vi "filter8.vi"(6 "initialize":bool, 8 "sampling freq: fs":dbl=1000.0 format="%#_13g", 9 "low cutoff freq: fl":dbl=30.0 format="%0.3f", 11 "X":dbl[](array[numeric])) -> (3 "Filtered X":dbl[](array[numeric]))   [LabVIEW 2016]
uses:
  <vilib>/imath/engines/lvmath2/RunTimeEngine/ErrorHandling/NIMS_Finalize Error.vi
  <vilib>/imath/engines/lvmath2/RunTimeEngine/NodeEndStatement/NIMS_NodeEndStatement_Output.vi
  <instcachedir>/0/NIMS_NodeEndStatement_Output_53EC0D466D134D7ABD903AC30B43404B.lvgen/NIMS_NodeEndStatement_Output_53EC0D466D134D7ABD903AC30B43404B_005.vi
  <vilib>/imath/engines/lvmath2/RunTimeEngine/BuiltInFunctions/double/NIMS_double.vi
  <instcachedir>/0/NIMS_double_34E32F64C2B04A25A042F4CA881A0A41.lvgen/NIMS_double_34E32F64C2B04A25A042F4CA881A0A41_002.vi
  <vilib>/ptbypt/NI_PtbyPt.lvlib
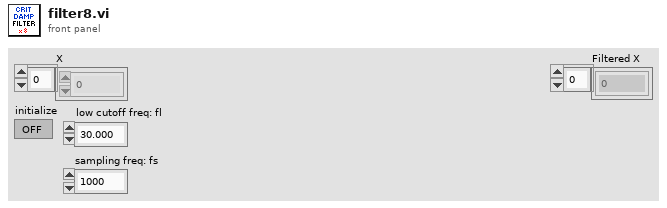
[diagram p1: front panel]
types:
  T1 = cluster{"filter structure":enum32{"IIR 2nd Order", "IIR 4th Order"}, "Reverse Coefficients":dbl[], "Forward Coefficients":dbl[]}
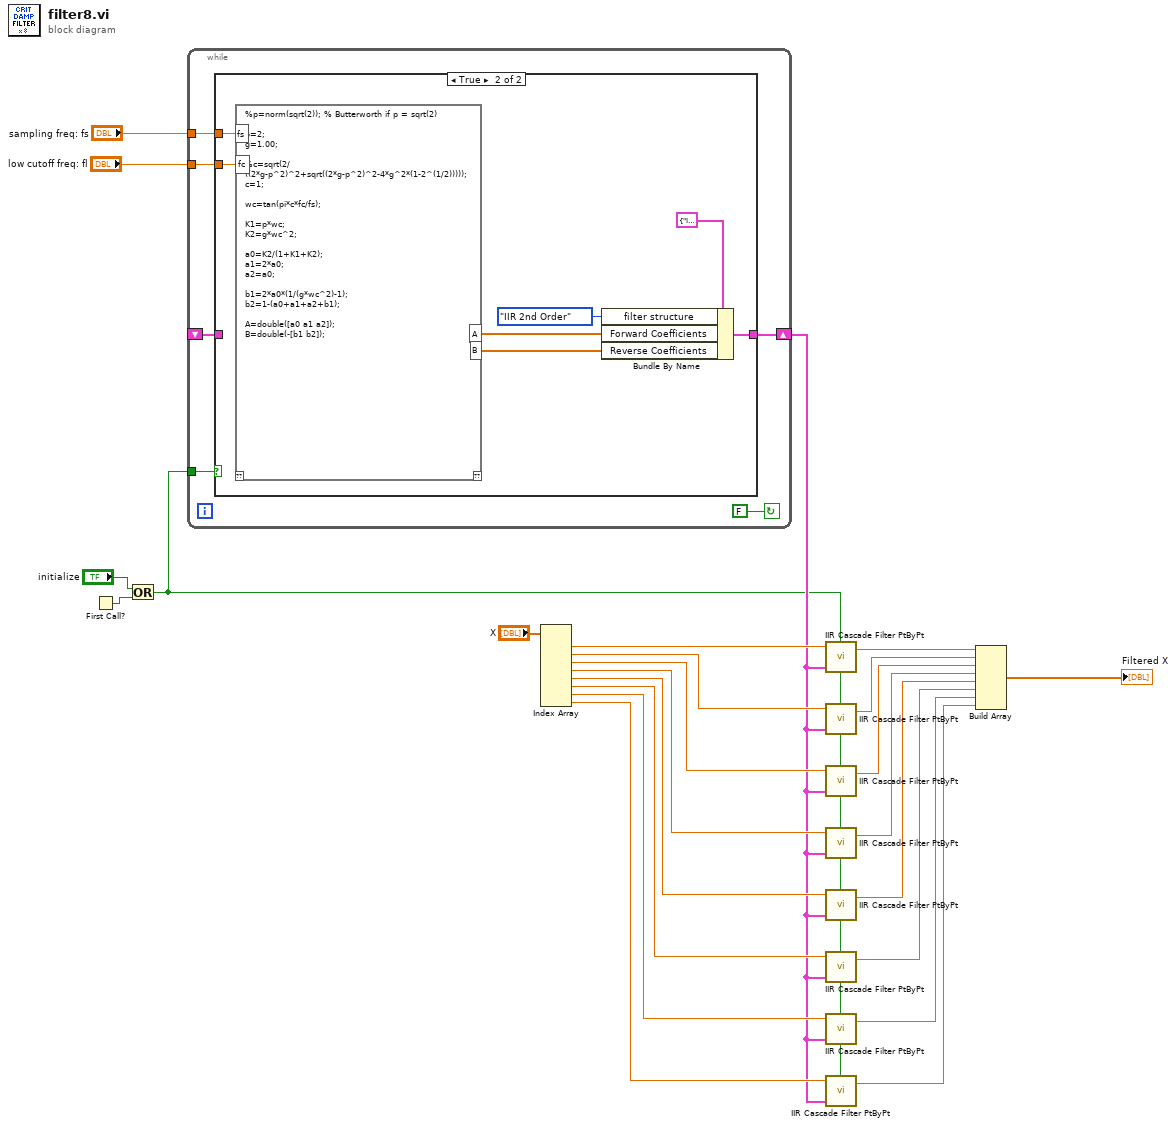
[diagram p0: block diagram]
diagram:
  n1 = First Call?() -> (First Call?: T/F=w3:bool)
  n2 = Or(x="initialize", y=w3) -> (x .or. y?=w1:bool)
  n3 = while {
    tunnel: "low cutoff freq: fl" -> [w29]
    tunnel: "sampling freq: fs" -> [w28]
    tunnel: w1 -> [w25]
    shift-right: [w30] -> w6
    shift-left: _ -> [w26]
    stop <- FALSE continue-if-true
    n4 = case shown="True" w25 {
      tunnel: [w31 w37] -> w30
      tunnel: w29 -> [_ w35]
      tunnel: w28 -> [_ w34]
      tunnel: w26 -> [w31 _]
      frame False {
      }
      frame True {
        n5 = mathscript code="%p=norm(sqrt(2)); % Butterworth if p = sqrt(2)\n\np=2;\ng=1.00;\n\n%c=sqrt(2/((2*g-p^2)^2+sqrt((2*g-p^2)^2-4*g^2*(1-2^(1/2)))));\nc=1;\n\nwc=tan(pi*c*fc/fs);\n\nK1=p*wc;\nK2=g*wc^2;\n\na0=K2/(1+K1+K2);\na1=2*a0;\na2=a0;\n\nb1=2*a0*(1/(g*wc^2)-1);\nb2=1-(a0+a1+a2+b1);\n\nA=double([a0 a1 a2]);\nB=double(-[b1 b2]);"("fs"=w34, "fc"=w35) -> ("A"=w33:dbl[], "B"=w32:dbl[])  [unwired: 1 in, 1 out]
        n6 = Bundle By Name(cluster=T1 {"filter structure"=enum."IIR 2nd Order", "Reverse Coefficients"=[], "Forward Coefficients"=[]} ("IIR Filter Cluster"), "filter structure"=enum32{"IIR 2nd Order", "IIR 4th Order"}."IIR 2nd Order", "Forward Coefficients"=w33, "Reverse Coefficients"=w32) -> (w37:T1)
      }
    }
  }
  n7 = Index Array(array="X") -> (element #1=w23:dbl, element #2=w22:dbl, element #3=w21:dbl, element #4=w20:dbl, element #5=w19:dbl, element #6=w18:dbl, element #7=w10:dbl, element #8=w8:dbl)  [unwired: 8 in]
  n8 = call <vilib>:"IIR Cascade Filter PtByPt.vi"("initialize"=w1, "IIR Filter Cluster"=w6, "x"=w23) -> ("Filtered x"=w17:dbl)  [unwired: 1 in, 1 out]
  n9 = call <vilib>:"IIR Cascade Filter PtByPt.vi"("initialize"=w1, "IIR Filter Cluster"=w6, "x"=w22) -> ("Filtered x"=w16:dbl)  [unwired: 1 in, 1 out]
  n10 = call <vilib>:"IIR Cascade Filter PtByPt.vi"("initialize"=w1, "IIR Filter Cluster"=w6, "x"=w21) -> ("Filtered x"=w15:dbl)  [unwired: 1 in, 1 out]
  n11 = call <vilib>:"IIR Cascade Filter PtByPt.vi"("initialize"=w1, "IIR Filter Cluster"=w6, "x"=w20) -> ("Filtered x"=w14:dbl)  [unwired: 1 in, 1 out]
  n12 = call <vilib>:"IIR Cascade Filter PtByPt.vi"("initialize"=w1, "IIR Filter Cluster"=w6, "x"=w19) -> ("Filtered x"=w13:dbl)  [unwired: 1 in, 1 out]
  n13 = call <vilib>:"IIR Cascade Filter PtByPt.vi"("initialize"=w1, "IIR Filter Cluster"=w6, "x"=w18) -> ("Filtered x"=w12:dbl)  [unwired: 1 in, 1 out]
  n14 = call <vilib>:"IIR Cascade Filter PtByPt.vi"("initialize"=w1, "IIR Filter Cluster"=w6, "x"=w10) -> ("Filtered x"=w11:dbl)  [unwired: 1 in, 1 out]
  n15 = call <vilib>:"IIR Cascade Filter PtByPt.vi"("initialize"=w1, "IIR Filter Cluster"=w6, "x"=w8) -> ("Filtered x"=w7:dbl)  [unwired: 1 in, 1 out]
  n16 = Build Array(w17, w16, w15, w14, w13, w12, w11, w7) -> (→"Filtered X":dbl[])
